vi "Cluster Ref.vi"(4 "Control Names to exlude":string[](array[string])=["error in (no error)", "error out", "Debug Abort"], 6 "Control State(Enable)":T1(ring), 8 "error in":errorcluster, 11 "Cluster Reference":refnum<vi>) -> (0 "error out":errorcluster)   [LabVIEW 2018]
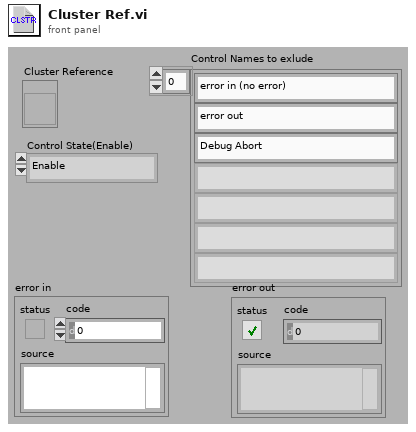
[diagram p1: front panel]
types:
  T1 = enum8{"Enable", "Disabled", "Disabled and Grayed"}
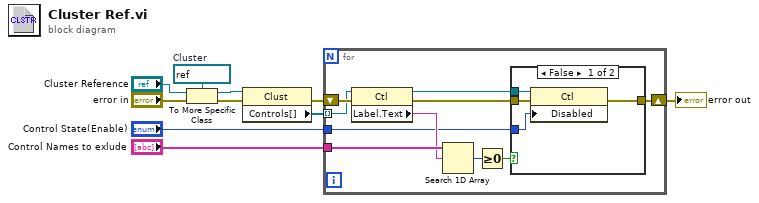
[diagram p0: block diagram]
diagram:
  w8 = refnum<vi> refnum  # Cluster
  n1 = To More Specific Class(target class=w8, reference="Cluster Reference", error in="error in") -> (specific class reference=w6:refnum<vi>, error out=w4:errorcluster)
  n2 = property class="Clust"(reference=w6, error in=w4) -> (error out=w10:errorcluster, "Controls[]"=w9:refnum<vi>[])  [unwired: 1 out]
  n3 = for {
    tunnel: w9 -> [w17] mode=indexing
    shift-right: [w15] -> w1
    shift-left: w10 -> [w20]
    tunnel: "Control Names to exlude" -> [w14]
    tunnel: "Control State(Enable)" -> [w12]
    n4 = property class="Ctl"(reference=w17, error in=w20) -> (reference out=w11:refnum<vi>, error out=w16:errorcluster, "Label.Text"=w13:string)
    n5 = Search 1D Array(1D array=w14, element=w13) -> (index of element=w19:i32)  [unwired: 1 out]
    n6 = Greater Or Equal To 0?(x=w19) -> (x >= 0?=w18:bool)
    n7 = case shown="False" w18 {
      tunnel: w16 -> [w24 w25]
      tunnel: [w22 w25] -> w15
      tunnel: w12 -> [w23 _]
      tunnel: w11 -> [w21 _]
      frame False {
        n8 = property class="Ctl"(reference=w21, error in=w24, "Disabled"=w23) -> (error out=w22:errorcluster)  [unwired: 1 out]
      }
      frame True {
      }
    }
  }
  "error out" <- w1
